vi "Actor Core.vi"(8 "error in":errorcluster, 11 "Duplicated Node Dialog View in":refnum<class "Duplicated Node Dialog View.lvclass">) -> (0 "error out":errorcluster, 3 "Actor out":refnum<class "Actor.lvclass">)   [LabVIEW 2013, in "Duplicated Node Dialog View.lvlib" / "Duplicated Node Dialog View.lvclass"]
doc: "(<B>Filename</B>: Actor Framework.lvlib:Actor.lvclass:Actor Core.vi)\n\nReceives messages to the actor, reacts to them, and initiates any error handling that may shut the actor down.\n\nDescendant classes may override this VI to append parallel tasks for the actor to complete while it handles messages. Overrides use the Call Parent Method node."
uses:
  Duplicated Node Dialog View.lvclass
  <vilib>/ActorFramework/Actor/Actor.lvclass
  Resources/UI Controls/Dark Theme/Push Button.ctl
  <vilib>/ActorFramework/Actor/Actor.lvclass/Actor.ctl
  <vilib>/ActorFrameworkMVC/View Actor/View Actor.lvclass
  <vilib>/Utility/miscctls.llb/LVPositionTypeDef.ctl
  <vilib>/ActorFrameworkMVC/UI Controller Messages/Move Subpanel Msg/Move Subpanel Msg.lvclass/Move Subpanel Msg.ctl
  <vilib>/ActorFramework/Message Enqueuer/Message Enqueuer.lvclass/Message Enqueuer.ctl
  <vilib>/ActorFramework/Message Enqueuer/Enqueue.vi
  <vilib>/ActorFramework/Message Priority Queue/Priority Enqueue.vi
  <vilib>/ActorFrameworkMVC/UI Controller Messages/Move Subpanel Msg/Move Subpanel Msg.lvclass
  Resources/UI Controls/Dark Theme/Dark Theme.lvlib
panel:
  in  "OK Button":T1
  out "Message":string="重复节点MAC配置，无法保存。"
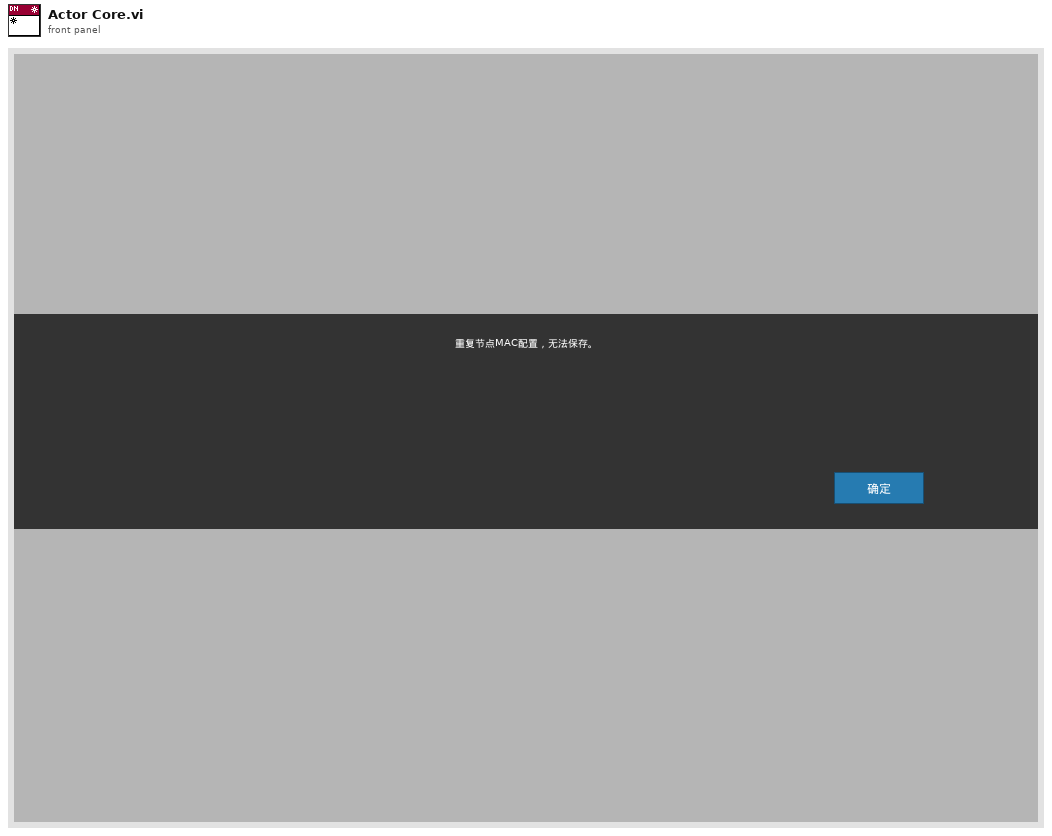
[diagram p1: front panel]
types:
  T1 = typedef "UI Control.lvlib/Dark Theme.lvlib/Push Button.ctl" = bool
  T2 = typedef "LVPositionTypeDef.ctl" = cluster{"Left":i32, "Top":i32}
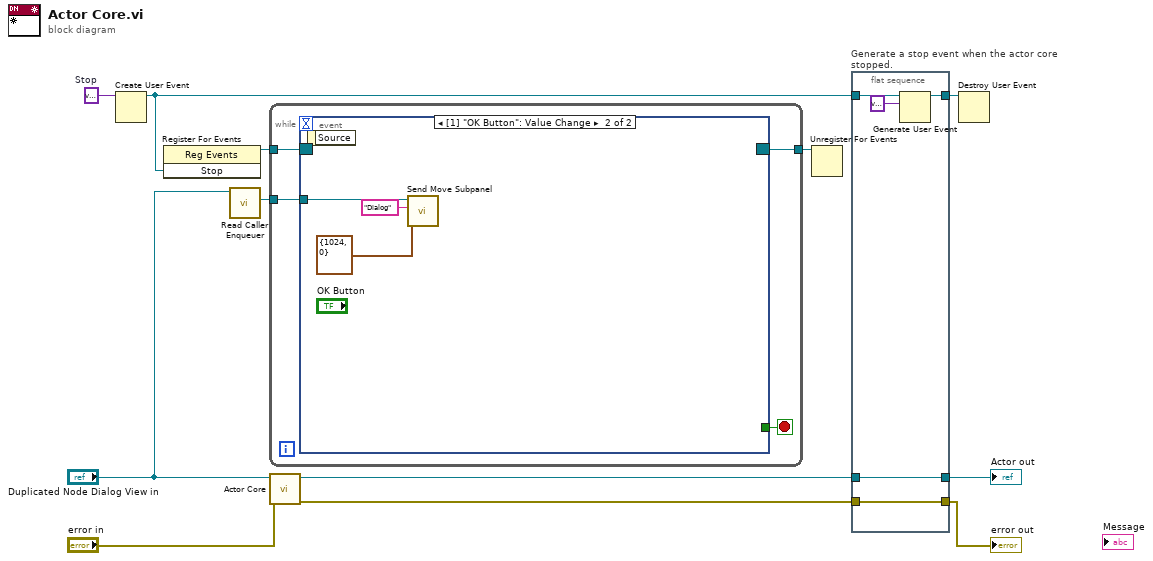
[diagram p0: block diagram]
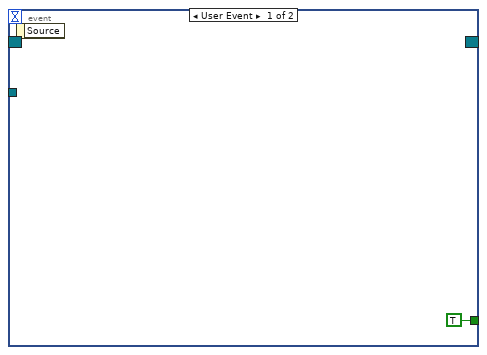
[diagram p2: hidden frame]
diagram:
  w12 = variant  # Stop
  n1 = Create User Event(user event datatype=w12) -> (user event=w4:refnum<user-event>)  [unwired: 1 in, 1 out]
  n2 = register-events(w4) -> (reference out=w5:refnum<event-registration>)  [unwired: 2 in, 1 out]
  n3 = call <vilib>:"Read Caller Enqueuer.vi"("Actor"="Duplicated Node Dialog View in") -> ("Caller Enqueuer"=w2:refnum<class "Message Enqueuer.lvclass">)  [unwired: 10 in]
  n4 = while {
    tunnel: [w16] -> w3
    tunnel: w5 -> [w14]
    tunnel: w2 -> [w13]
    stop <- w15 stop-if-true
    n5 = event shown="[1] \"OK Button\": Value Change" {
      selector: w14 -> [_ _]
      dyn-events: [_ _] -> w16
      timeout: _ -> [_ _]
      tunnel: [TRUE _] -> w15
      tunnel: w13 -> [_ w20]
      event User Event {
        n6 = event-data() -> ()  [unwired: 1 in, 1 out]
      }
      event Value Change {
        n7 = event-data() -> ()  [unwired: 1 in, 1 out]
        n8 = call <vilib>:"Send Move Subpanel.vi"("Position (0,0)"=T2 {"Left"=1024, "Top"=0}, "Subpanel Name"="Dialog", "Message Enqueuer"=w20) -> ()  [unwired: 7 in, 2 out]
      }
    }
  }
  n9 = call-parent "Actor Core.vi"("error in"="error in", "View Actor in"="Duplicated Node Dialog View in") -> ("error out"=w8:errorcluster, "Actor out"=w9:refnum<class "Actor.lvclass">)  [unwired: 8 in]
  n10 = Unregister For Events(event registration refnum=w3) -> ()  [unwired: 1 in, 1 out]
  n11 = flat-sequence "Generate a stop event when the actor core stopped." {
    tunnel: w4 -> [w25]
    tunnel: [w23] -> w11
    tunnel: w9 -> [w22]
    tunnel: w8 -> [w21]
    tunnel: [w22] -> w7
    tunnel: [w21] -> w6
    frame #0 {
      n12 = Generate User Event(user event=w25, event data cluster=variant ("event data")) -> (user event out=w23:refnum<user-event>)  [unwired: 2 in, 1 out]
    }
  }
  n13 = Destroy User Event(user event=w11) -> ()  [unwired: 1 in, 1 out]
  "error out" <- w6
  "Actor out" <- w7
